vi "WriteHooverOverInfo.vi"(8 "error in (no error)":errorcluster, 10 "HooverOverInfo":string, 11 "Parameter In":refnum<class "Parameter.lvclass">) -> (0 "error out":errorcluster, 3 "Parameter out":refnum<class "Parameter.lvclass">)   [LabVIEW 2023, in "Easy.SequenceManagerLabVIEW.lvlib" / "Parameter.lvclass"]
uses:
  Parameter.lvclass
  Parameter.lvclass/Parameter.ctl
panel:
  # "Connector Pane"
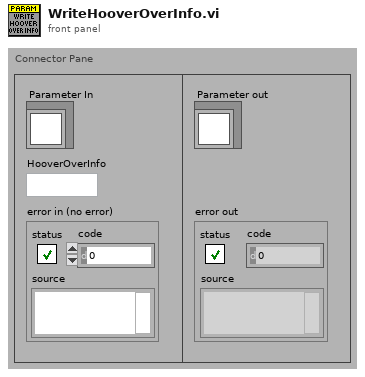
[diagram p1: front panel]
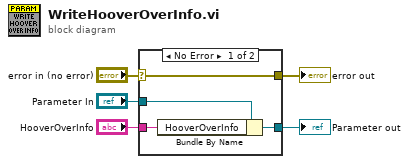
[diagram p0: block diagram]
diagram:
  n1 = case shown="No Error" "error in (no error)" {
    selector: "error in (no error)" -> [w8 w11]
    tunnel: [w8 w11] -> w4
    tunnel: [w6 w10] -> w2
    tunnel: "Parameter In" -> [w7 w10]
    tunnel: "HooverOverInfo" -> [w9 _]
    frame No Error {
      n2 = Bundle By Name(cluster=w7, "HooverOverInfo"=w9) -> (w6:refnum<class "Parameter.lvclass">)
    }
    frame Error {
    }
  }
  "error out" <- w4
  "Parameter out" <- w2
